vi "onMouseEnter.vi"(8 "error in (no error)":errorcluster, 11 "Filled Text Fields Actor in":refnum<class "Filled Text Fields Actor.lvclass">) -> (0 "error out":errorcluster, 3 "Filled Text Fields Actor out":refnum<class "Filled Text Fields Actor.lvclass">)   [LabVIEW 2017, in "Filled Text Fields.lvlib" / "Filled Text Fields Actor.lvclass"]
uses:
  Filled Text Fields Actor.lvclass
  Filled Text Fields Actor.lvclass/Filled Text Fields Actor.ctl
  Filled Text Fields.States.ctl
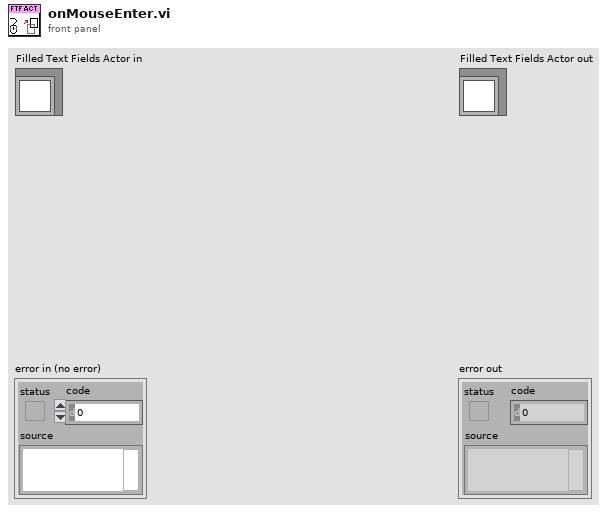
[diagram p1: front panel]
types:
  T1 = typedef "Filled Text Fields.lvlib/Filled Text Fields Actor.lvclass/Filled Text Fields.States.ctl" = enum16{"Inactive", "Activated", "Error", "Focused", "Hover", "Disabled", "Disabled and Grey out"}
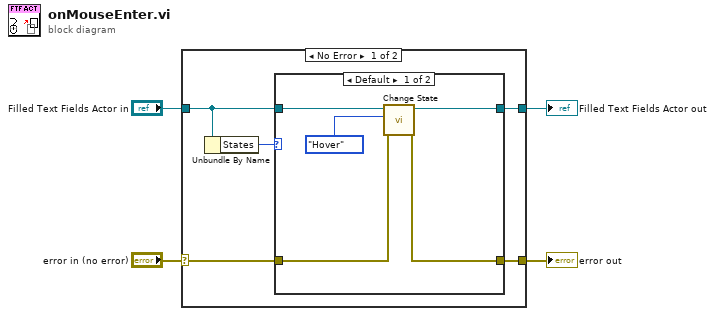
[diagram p0: block diagram]
diagram:
  n1 = case shown="No Error" "error in (no error)" {
    selector: "error in (no error)" -> [w8 w18]
    tunnel: [w7 w18] -> w3
    tunnel: [w9 w17] -> w1
    tunnel: "Filled Text Fields Actor in" -> [w6 w17]
    frame No Error {
      n2 = Unbundle By Name(w6) -> ("States"=w5:T1)
      n3 = case shown="Default" w5 {
        tunnel: [w14 w16] -> w9
        tunnel: w8 -> [w13 w15]
        tunnel: [w12 w15] -> w7
        tunnel: w6 -> [w10 w16]
        frame Default {
          n4 = call "Change State.vi"("error in (no error)"=w13, "New State"=Filled_Text_Fields.States."Hover", "Filled Text Fields Actor in"=w10) -> ("error out"=w12:errorcluster, "Filled Text Fields Actor out"=w14:refnum<class "Filled Text Fields Actor.lvclass">)  [unwired: 7 in]
        }
        frame "Focused" {
        }
      }
    }
    frame Error {
    }
  }
  "error out" <- w3
  "Filled Text Fields Actor out" <- w1
